vi "Upload OD Entries.vi"(8 "error in":errorcluster, 10 "Entries":refnum<class "OD Entry.lvclass">[](array[class]), 11 "Interactor in":refnum<class "Interactor.lvclass">) -> (0 "error out":errorcluster, 2 "Values":T1(array[cluster]) {"Multiplexer"."Index" format="%.0x"}, 3 "Interactor out":refnum<class "Interactor.lvclass">)   [LabVIEW 2020, in "Interactor.lvlib" / "Interactor.lvclass"]
uses:
  Interactor.lvclass
  Interactor.lvclass/Interactor.ctl
  CANopen Master/CANopen Master.lvclass
  EDS-File-Viewer/source/Core/OD Entry/OD Entry.lvclass
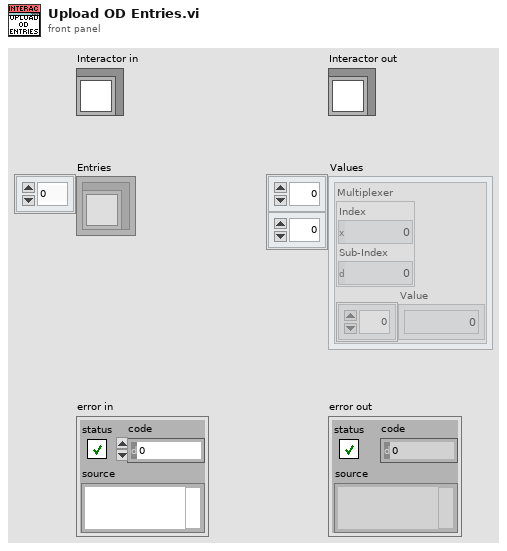
[diagram p1: front panel]
types:
  T1 = cluster{"Multiplexer":cluster{"Index":u16, "Sub-Index":i16}, "Value":u8[]}[][]
  T2 = cluster{"Multiplexer":cluster{"Index":u16, "Sub-Index":i16}, "Value":u8[]}
  T3 = cluster{"Multiplexer":cluster{"Index":u16, "Sub-Index":i16}, "Value":u8[]}[]
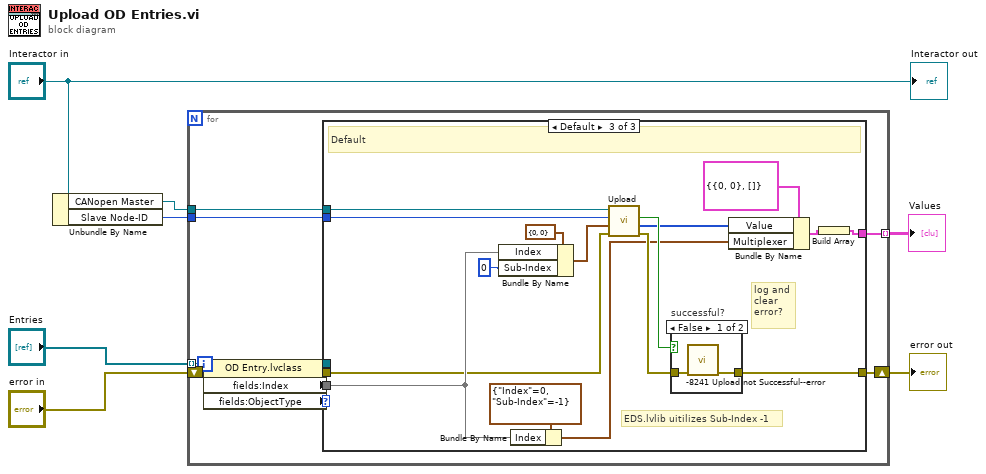
[diagram p0: block diagram]
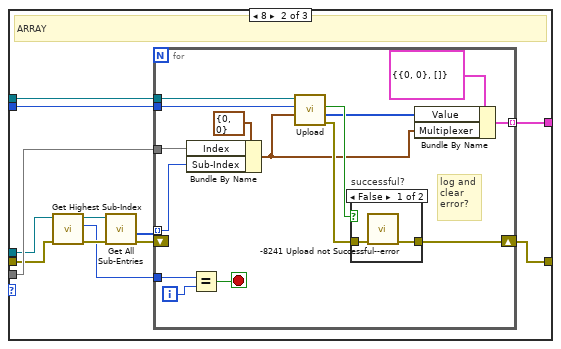
[diagram p3: hidden frame]
diagram:
  n1 = Unbundle By Name("Interactor in") -> ("CANopen Master"=w5:refnum<class "CANopen Master.lvclass">, "Slave Node-ID"=w4:u8)
  n2 = for {
    tunnel: "Entries" -> [w12] mode=indexing
    tunnel: w5 -> [w17]
    tunnel: w4 -> [w16]
    shift-right: [w14] -> w2
    shift-left: "error in" -> [w15]
    tunnel: [w13] -> w1 mode=indexing
    n3 = property class="OD Entry.lvclass"(reference=w12, error in=w15) -> (reference out=w8:refnum<class "OD Entry.lvclass">, error out=w11:errorcluster, "fields:Index"=w10, "fields:ObjectType"=w9)
    n4 = case shown="Default" w9 {
      tunnel: w17 -> [_ w30 w64]
      tunnel: w16 -> [_ w29 w63]
      tunnel: [w18 w28 w62] -> w14
      tunnel: [_ w27 w54] -> w13
      tunnel: w11 -> [w18 w23 w49]
      tunnel: w10 -> [_ w26 w52]
      tunnel: w8 -> [_ w21 _]
      frame 9 {
        # "RECORD"
      }
      frame 8 {
        # "ARRAY"
        n5 = call "Get Highest Sub-Index.vi"("Error In"=w23, "reference in"=w21) -> ("Error Out"=w22:errorcluster, "Highest Sub-Index"=w19:i16, "reference out"=w20:refnum<class "OD Entry.lvclass">)  [unwired: 7 in]
        n6 = call "Get All Sub-Entries.vi"("Error In"=w22, "reference in"=w20) -> ("Error Out"=w25:errorcluster, "Indices"=w24:u8[])  [unwired: 6 in, 2 out]
        n7 = for {
          tunnel: w26 -> [w36]
          tunnel: w30 -> [w45]
          tunnel: w29 -> [w44]
          tunnel: [w42] -> w27 mode=indexing
          shift-right: [w41] -> w28
          shift-left: w25 -> [_]
          tunnel: w24 -> [w32] mode=indexing
          tunnel: w19 -> [w33]
          i -> [w35]
          stop <- w34 stop-if-true
          # "log and\nclear\nerror?"
          n8 = Bundle By Name(cluster=cluster{"Index":u16, "Sub-Index":u8} {"Index"=0, "Sub-Index"=0} ("Multiplexer"), "Index"=w36, "Sub-Index"=w32) -> (w31:cluster{"Index":u16, "Sub-Index":u8})
          n9 = Equal?(x=w33, y=w35) -> (x = y?=w34:bool)
          n10 = call "Upload.vi"("Multiplexer"=w31, "Node-ID"=w44, "CANopen Master in"=w45) -> ("error out"=w40:errorcluster, "Value"=w37:u8[], "Success?"=w39:bool)  [unwired: 5 in, 1 out]
          n11 = case "successful?" shown="False" w39 {
            tunnel: w40 -> [w47 w48]
            tunnel: [w46 w48] -> w41
            frame False {
              n12 = call "-8241 Upload not Successful--error.vi"("error in"=w47) -> ("error out"=w46:errorcluster)  [unwired: 10 in]
            }
            frame True {
            }
          }
          n13 = Bundle By Name(cluster=T2 {"Multiplexer"={"Index"=0, "Sub-Index"=0}, "Value"=[]}, "Value"=w37, "Multiplexer"=w31) -> (w42:T2)
        }
      }
      frame Default {
        # "EDS.lvlib uitilizes Sub-Index -1"
        # "log and\nclear\nerror?"
        # "Default"
        n14 = Bundle By Name(cluster=cluster{"Index":u16, "Sub-Index":u8} {"Index"=0, "Sub-Index"=0} ("Multiplexer"), "Index"=w52, "Sub-Index"=u8 0) -> (w50:cluster{"Index":u16, "Sub-Index":u8})
        n15 = Bundle By Name(cluster=cluster{"Index":u16, "Sub-Index":i16} {"Index"=0, "Sub-Index"=-1} ("Multiplexer"), "Index"=w52) -> (w55:cluster{"Index":u16, "Sub-Index":i16})
        n16 = call "Upload.vi"("error in"=w49, "Multiplexer"=w50, "Node-ID"=w63, "CANopen Master in"=w64) -> ("error out"=w59:errorcluster, "Value"=w56:u8[], "Success?"=w58:bool)  [unwired: 4 in, 1 out]
        n17 = case "successful?" shown="False" w58 {
          tunnel: w59 -> [w66 w67]
          tunnel: [w65 w67] -> w62
          frame False {
            n18 = call "-8241 Upload not Successful--error.vi"("error in"=w66) -> ("error out"=w65:errorcluster)  [unwired: 10 in]
          }
          frame True {
          }
        }
        n19 = Bundle By Name(cluster=T2 {"Multiplexer"={"Index"=0, "Sub-Index"=0}, "Value"=[]}, "Value"=w56, "Multiplexer"=w55) -> (w61:T2)
        n20 = Build Array(w61) -> (w54:T3)
      }
    }
  }
  "error out" <- w2
  "Values" <- w1
  "Interactor out" <- "Interactor in"
